vi "PipBoy_SetPageNum.vi"(8 "error in (no error)":errorcluster, 9 "PageTot":i32, 10 "PageNum":i32, 11 "VisaPic32In":refnum<visa-resource-name>) -> (0 "error out":errorcluster, 3 "VisaPic32Out":refnum<visa-resource-name>)   [LabVIEW 2014]
uses:
  <vilib>/Utility/error.llb/Error Cluster From Error Code.vi
  <vilib>/ErrorRing/Error Ring.xnode
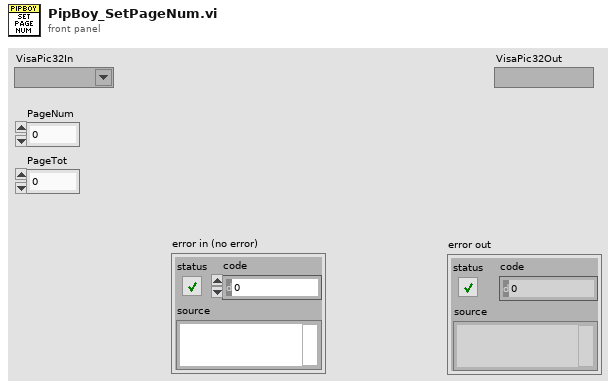
[diagram p1: front panel]
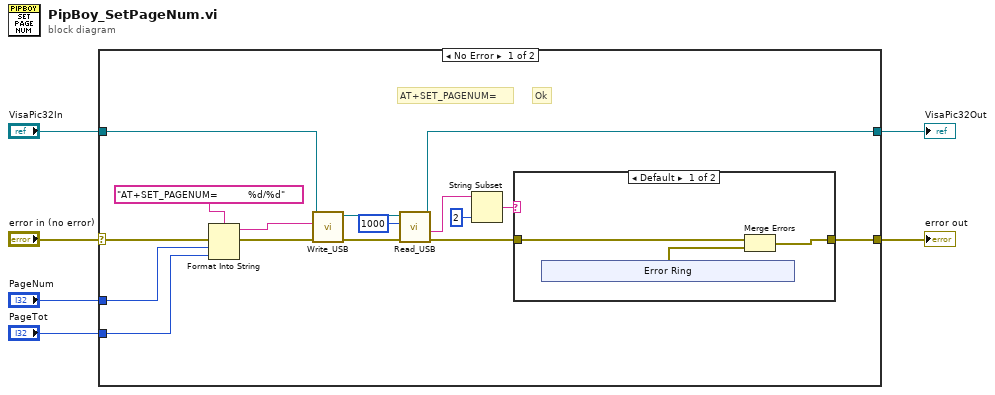
[diagram p0: block diagram]
diagram:
  n1 = case shown="No Error" "error in (no error)" {
    selector: "error in (no error)" -> [w15 w33]
    tunnel: [w17 w33] -> w5
    tunnel: "VisaPic32In" -> [w19 w32]
    tunnel: [w16 w32] -> w3
    tunnel: "PageNum" -> [w11 _]
    tunnel: "PageTot" -> [w10 _]
    frame No Error {
      # "Ok"
      # "AT+SET_PAGENUM="
      n2 = Format Into String(format string="AT+SET_PAGENUM=          %d/%d" ("buffer d'écriture"), error in=w15, w11, w10) -> (resulting string=w12:string, error out=w14:errorcluster)  [unwired: 1 in]
      n3 = call "Write_USB.vi"("entrée d'erreur"=w14, "buffer d'écriture"=w12, "Nom de ressource VISA"=w19) -> ("sortie d'erreur"=w22:errorcluster, "Nom de ressource VISA en sortie"=w21:refnum<visa-resource-name>)  [unwired: 7 in]
      n4 = call "Read_USB.vi"("entrée d'erreur"=w22, "timeout (0)"=u32 1000, "Nom de ressource VISA"=w21) -> ("sortie d'erreur"=w18:errorcluster, "chaîne en sortie"=w8:string, "Nom de ressource VISA en sortie"=w16:refnum<visa-resource-name>)  [unwired: 6 in]
      n5 = String Subset(string=w8, length (rest)=2 ("length (rest)")) -> (substring=w7:string)  [unwired: 1 in]
      n6 = case shown="Default" w7 {
        tunnel: [w24 w31] -> w17
        tunnel: w18 -> [w25 w31]
        frame Default {
          n7 = xnode "Error Ring"() -> ("error out"=w23:errorcluster)
          n8 = Merge Errors(w25, w23) -> (w24:errorcluster)
        }
        frame "OK" {
        }
      }
    }
    frame Error {
    }
  }
  "error out" <- w5
  "VisaPic32Out" <- w3
